vi "2D Cartesian Coordinate Rotation.vi"   [LabVIEW 2012, in "NI_AALPro.lvlib"]
doc: "Rotates a two-dimensional Cartesian coordinate system in the counterclockwise direction. Wire data to the <B>X</B> input to determine the polymorphic instance to use or manually select the instance."
uses:
  NI_AALPro.lvlib
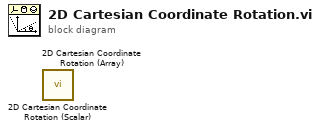
[diagram p0: block diagram]
diagram:
  n1 = call "2D Cartesian Coordinate Rotation (Scalar).vi"() -> ()  [unwired: 9 in, 3 out]
  n2 = call "2D Cartesian Coordinate Rotation (Array).vi"() -> ()  [unwired: 9 in, 3 out]
